vi "Load-deposition-files.vi"(8 "error in (no error)":errorcluster, 11 "Object ref in":T1) -> (0 "error out":errorcluster, 3 "Object ref out":T1)   [LabVIEW 2013, in "SLMControl.lvlib" / "SC-Main.lvclass"]
uses:
  SC-Main.lvclass
  Object-reference.ctl
  SC-Main.lvclass/SC-Main.ctl
  UI/Control-names.ctl
  Application-status.ctl
  Read UI.vi
  Read Lasing files.vi
  Read Status.vi
  Read Base path.vi
  UI/Set-control-boolean.vi
  UI/Set-control-enable-single.vi
  UI/SC-UI.lvclass
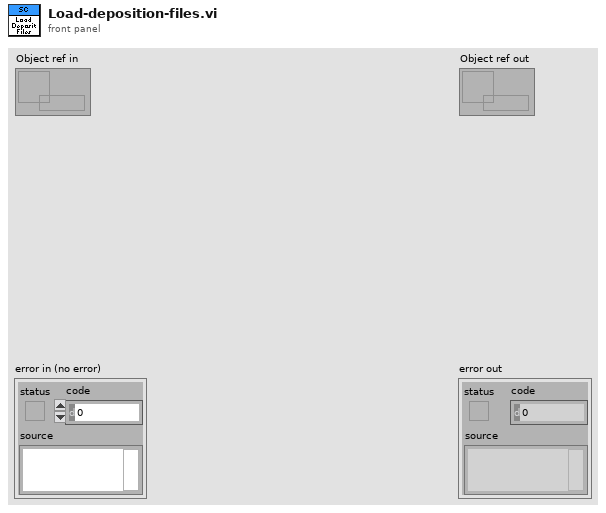
[diagram p1: front panel]
types:
  T1 = typedef "SLMControl.lvlib/SC-Main.lvclass/Object-reference.ctl" = refnum<data-value>
  T2 = typedef "SLMControl.lvlib/SC-UI.lvclass/Control-names.ctl" = enum16{"Com-in", "Com-out", "Help", "Status", "Load configuration", "Save configuration", "Load lasing files", "Load deposition files", "Clear", "Files", "Activate", "Execute", "Abort", "Options", "Current layer", "Current iteration", "Last elapsed time", "Deposition status", "Lasing job", "Status LEDs", "Exiting led", "Initialized led", "Files loaded led", "Activated led", "Executing led", "Deposition led", "Lasing job led", "Lasing led"}
  T3 = typedef "SLMControl.lvlib/SC-Main.lvclass/Application-status.ctl" = enum16{"Idle", "Initialized", "Configured", "Activated", "Started", "Paused", "Stopped", "Reset", "Error", "Exited"}
  T4 = typedef "SLMControl.lvlib/SC-UI.lvclass/Panes-reference.ctl" = refnum<data-value>
  T5 = typedef "SLMControl.lvlib/SC-Main.lvclass/Client-status.ctl" = enum16{"Idle", "Initialized", "Configured", "Activated", "Started", "Paused", "Stopped", "Reset", "Error", "Exited"}
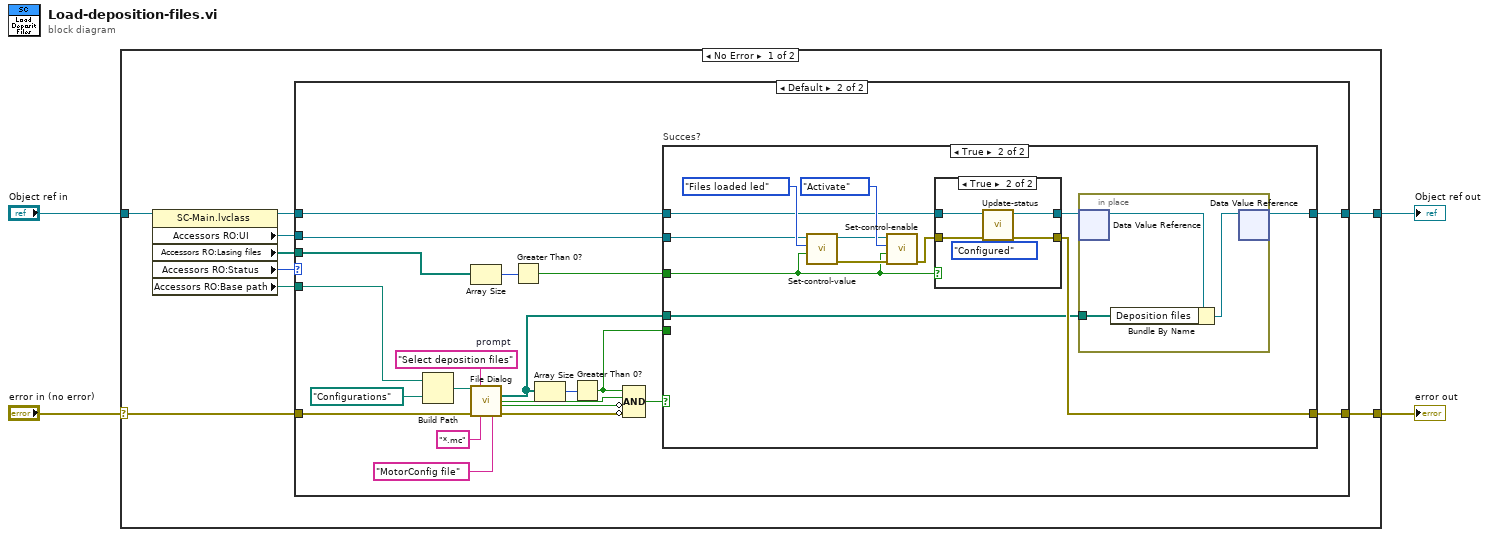
[diagram p0: block diagram]
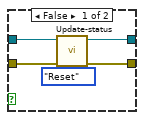
[diagram p4: hidden frame]
diagram:
  n1 = case shown="No Error" "error in (no error)" {
    selector: "error in (no error)" -> [w13 w64]
    tunnel: [w8 w64] -> w3
    tunnel: [w7 w63] -> w1
    tunnel: "Object ref in" -> [w12 w63]
    frame No Error {
      n2 = property class="SC-Main.lvclass"(reference=w12) -> (reference out=w9:T1, "Accessors RO:UI"=w10:T4, "Accessors RO:Lasing files"=w11:path[], "Accessors RO:Status"=w6:T5, "Accessors RO:Base path"=w5:path)  [unwired: 1 in, 1 out]
      n3 = case shown="Default" w6 {
        tunnel: w13 -> [w15 w34]
        tunnel: w11 -> [_ w29]
        tunnel: w10 -> [_ w19]
        tunnel: w9 -> [w14 w26]
        tunnel: [w15 w24] -> w8
        tunnel: [w14 w23] -> w7
        tunnel: w5 -> [_ w16]
        frame "Activated".."Paused" {
        }
        frame Default {
          w36 = "Select deposition files"  # prompt
          n4 = Build Path(base path=w16, name or relative path=path "Configurations") -> (appended path=w17:path)
          n5 = Array Size(array=w29) -> (size(s)=w28:i32)
          n6 = call "File Dialog"("start path"=w17, "prompt"=w36, "error in"=w34, "pattern (all files)"="*.mc", "pattern label"="MotorConfig file") -> ("selected paths"=w25:path[], "exists"=w31:bool, "cancelled"=w30:bool, "error out"=w27:errorcluster)  [unwired: 7 in]
          n7 = Greater Than 0?(x=w28) -> (x > 0?=w20:bool)
          n8 = Array Size(array=w25) -> (size(s)=w32:i32)
          n9 = Greater Than 0?(x=w32) -> (x > 0?=w22:bool)
          n10 = Compound Arithmetic op=AND(w22, w31, invert w30, invert w27) -> (w21:bool)
          n11 = case "Succes?" shown="True" w21 {
            tunnel: [_ w49] -> w24
            tunnel: [w37 w47] -> w23
            tunnel: w19 -> [_ w39]
            tunnel: w26 -> [w37 w40]
            tunnel: w25 -> [_ w46]
            tunnel: w22 -> [_ _]
            tunnel: w20 -> [_ w38]
            frame False {
            }
            frame True {
              n12 = call-poly "Set-control-value.vi"("Value"=w38, "Control name"=Control-names."Files loaded led", "Panes in"=w39) -> ("error out"=w43:errorcluster, "Panes out"=w44:T4)  [unwired: 7 in]
              n13 = call-poly "Set-control-enable.vi"("error in (no error)"=w43, "Enable?"=w38, "Control name"=Control-names."Activate", "Panes in"=w44) -> ("error out"=w41:errorcluster)  [unwired: 6 in, 1 out]
              n14 = case shown="True" w38 {
                tunnel: [w51 w59] -> w49
                tunnel: [w50 w57] -> w48
                tunnel: w41 -> [w52 w56]
                tunnel: w40 -> [w53 w55]
                frame False {
                  n15 = call "Update-status.vi"("Status"=Application-status."Reset", "error in (no error)"=w52, "Object ref in"=w53) -> ("error out"=w51:errorcluster, "Object ref out"=w50:T1)  [unwired: 7 in]
                }
                frame True {
                  n16 = call "Update-status.vi"("Status"=Application-status."Configured", "error in (no error)"=w56, "Object ref in"=w55) -> ("error out"=w59:errorcluster, "Object ref out"=w57:T1)  [unwired: 7 in]
                }
              }
              n17 = in-place {
                in-place-border: w46 -> [w61]
                n18 = in-place-dvr #1(w48) -> (w62:refnum<class "SC-Main.lvclass">)  [unwired: 1 out]
                n19 = Bundle By Name(cluster=w62, "Deposition files"=w61) -> (w60:refnum<class "SC-Main.lvclass">)
                n20 = in-place-dvr #1(w60) -> (w47:T1)  [unwired: 1 out]
              }
            }
          }
        }
      }
    }
    frame Error {
    }
  }
  "error out" <- w3
  "Object ref out" <- w1
